vi "write slope info to clusters.vi"(0 "DHT_Pressure_ Offset":dbl, 1 "DHT_Pressure Slope":dbl, 2 "Output Slopes Cluster in":T1, 3 "Input Variables and Slopes in":T2 {"Feet of Stainless" format="%.2f"; "Height of Sample Box" format="%.2f"; "Reservoir Pressure" format="%.2f"; "Flow Offset" format="%.2f"; "String Pot Offset" format="%.2f"; "Aux 3 Offset" format="%.2f"; "Aux 2 Offset" format="%.2f"; "Aux 1 Offset" format="%.2f"; "Aux 3 Slope" format="%.2f"; "Aux 2 Slope" format="%.2f"; "Aux 1 Slope" format="%.2f"; "Up Hole  Pressure Offset" format="%.2f"; "DH Pressure Offset" format="%.2f"; "DH Pressure Trans Slope" format="%.2f"; "Atmospheric Pressure" format="%.2f"; "Depth to Water Table" format="%.2f"; "Up Hole Pressure Slope" format="%.2f"; "Flow Slope" format="%.2f"; "String Pot Slope" format="%.2f"; "Total Volume" format="%.2f"}, 5 "Aux1_Slope In":dbl, 7 "pressure_slope_IN":dbl, 9 "Aux2_Slope In":dbl, 12 "Aux3_ Slope In":dbl, 13 "string_pot_slope_IN":dbl, 14 "flow_slope_IN":dbl) -> (4 "Input Variables and Slopes out":T2 {"Feet of Stainless" format="%.2f"; "Height of Sample Box" format="%.2f"; "Reservoir Pressure" format="%.2f"; "Flow Offset" format="%.2f"; "String Pot Offset" format="%.2f"; "Aux 3 Offset" format="%.2f"; "Aux 2 Offset" format="%.2f"; "Aux 1 Offset" format="%.2f"; "Aux 3 Slope" format="%.2f"; "Aux 2 Slope" format="%.2f"; "Aux 1 Slope" format="%.2f"; "Up Hole  Pressure Offset" format="%.2f"; "DH Pressure Offset" format="%.2f"; "DH Pressure Trans Slope" format="%.2f"; "Atmospheric Pressure" format="%.2f"; "Depth to Water Table" format="%.2f"; "Up Hole Pressure Slope" format="%.2f"; "Flow Slope" format="%.2f"; "String Pot Slope" format="%.2f"; "Total Volume" format="%.2f"}, 6 "Output Slopes Cluster out":T1)   [LabVIEW 2016]
uses:
  KPRO_2016 subvis/Control 2.ctl
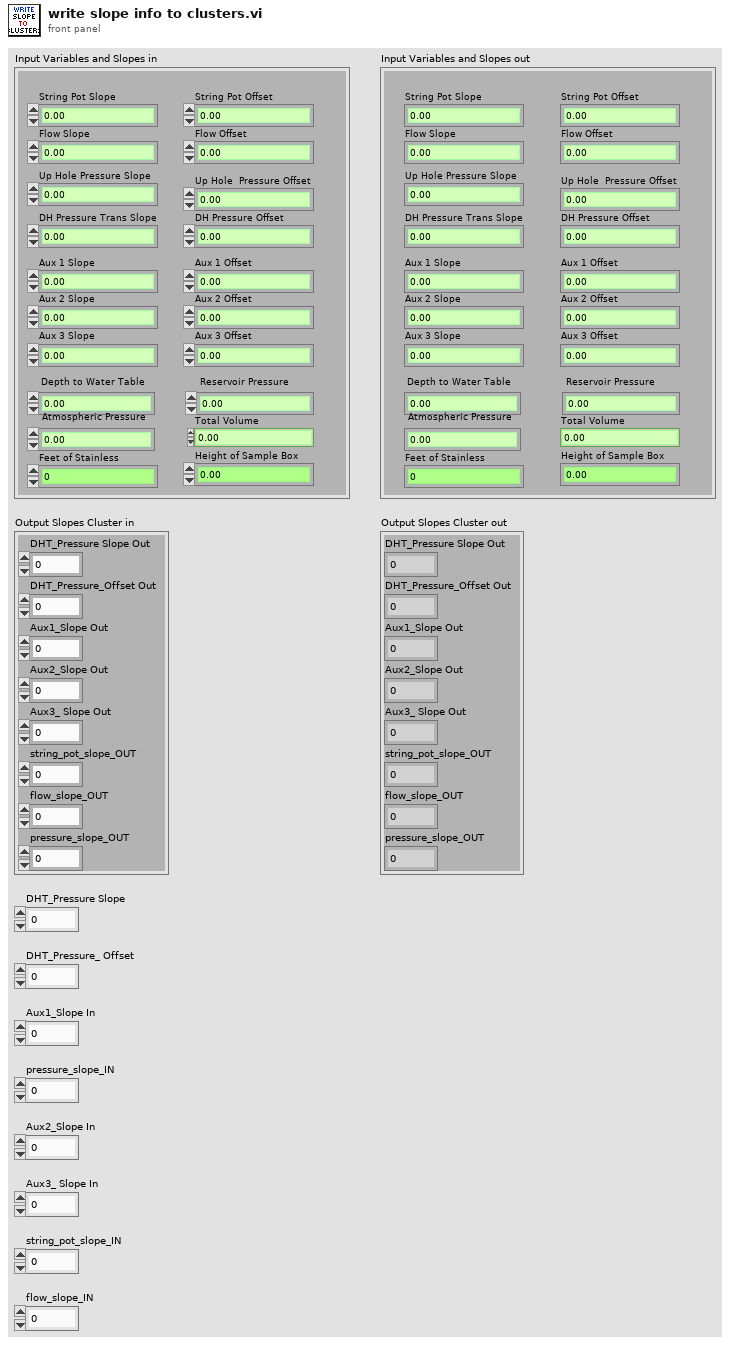
[diagram p1: front panel]
types:
  T1 = cluster{"DHT_Pressure Slope Out":dbl, "DHT_Pressure_Offset Out":dbl, "Aux1_Slope Out":dbl, "Aux2_Slope Out":dbl, "Aux3_ Slope Out":dbl, "string_pot_slope_OUT":dbl, "flow_slope_OUT":dbl, "pressure_slope_OUT":dbl}
  T2 = typedef "Control 2.ctl" = cluster{"Total Volume":dbl, "String Pot Slope":dbl, "Flow Slope":dbl, "Up Hole Pressure Slope":dbl, "Depth to Water Table":dbl, "Atmospheric Pressure":dbl, "DH Pressure Trans Slope":dbl, "DH Pressure Offset":dbl, "Up Hole  Pressure Offset":dbl, "Aux 1 Slope":dbl, "Aux 2 Slope":dbl, "Aux 3 Slope":dbl, "Aux 1 Offset":dbl, "Aux 2 Offset":dbl, "Aux 3 Offset":dbl, "String Pot Offset":dbl, "Flow Offset":dbl, "Reservoir Pressure":dbl, "Height of Sample Box":dbl, "Feet of Stainless ":i32}
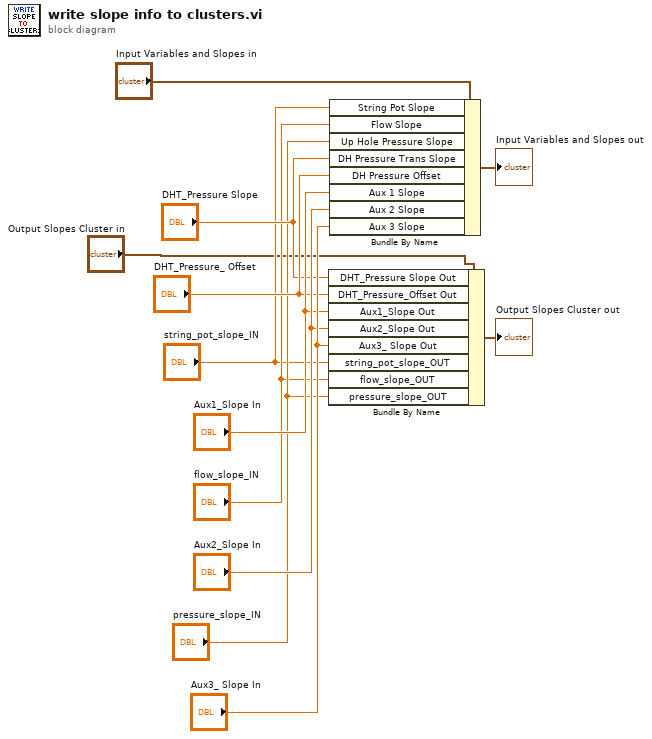
[diagram p0: block diagram]
diagram:
  n1 = Bundle By Name(cluster="Output Slopes Cluster in", "DHT_Pressure Slope Out"="DHT_Pressure Slope", "DHT_Pressure_Offset Out"="DHT_Pressure_ Offset", "Aux1_Slope Out"="Aux1_Slope In", "Aux2_Slope Out"="Aux2_Slope In", "Aux3_ Slope Out"="Aux3_ Slope In", "string_pot_slope_OUT"="string_pot_slope_IN", "flow_slope_OUT"="flow_slope_IN", "pressure_slope_OUT"="pressure_slope_IN") -> (→"Output Slopes Cluster out":T1)
  n2 = Bundle By Name(cluster="Input Variables and Slopes in", "String Pot Slope"="string_pot_slope_IN", "Flow Slope"="flow_slope_IN", "Up Hole Pressure Slope"="pressure_slope_IN", "DH Pressure Trans Slope"="DHT_Pressure Slope", "DH Pressure Offset"="DHT_Pressure_ Offset", "Aux 1 Slope"="Aux1_Slope In", "Aux 2 Slope"="Aux2_Slope In", "Aux 3 Slope"="Aux3_ Slope In") -> (→"Input Variables and Slopes out":T2)
